vi "Does the Text Fit.vi"(0 "user-specified font":T1, 5 "token string":string, 7 "Capitalize Text":bool) -> (4 "Text Fits":bool)   [LabVIEW 2020, in "Text-Based VI Icon.lvlib"]
uses:
  <vilib>/LabVIEW Icon API/Set Text Icon/Text-Based VI Icon.lvlib
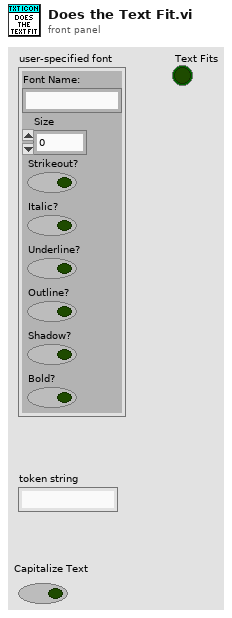
[diagram p1: front panel]
types:
  T1 = cluster{"Font Name:":string, "Size":i16, "Strikeout?":bool, "Italic?":bool, "Underline?":bool, "Outline?":bool, "Shadow?":bool, "Bold?":bool}
  T2 = enum16{"User-specified Font", "Application Font", "System Font", "Dialog Font"}
  T3 = cluster{"left":i16, "top":i16, "right":i16, "bottom":i16}
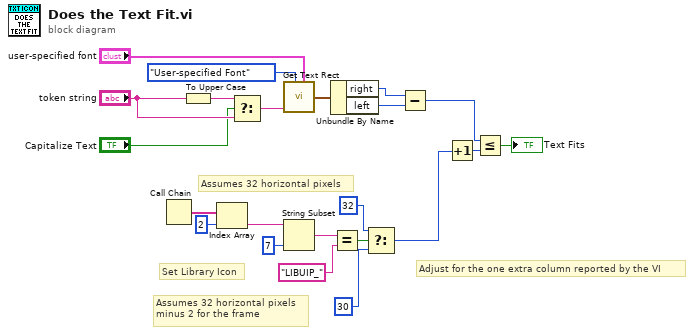
[diagram p0: block diagram]
diagram:
  # "Assumes 32 horizontal pixels\nminus 2 for the frame"
  # "Assumes 32 horizontal pixels"
  # "Set Library Icon"
  # "Adjust for the one extra column reported by the VI"
  n1 = Call Chain() -> (call chain=w10:string[])
  n2 = To Upper Case(1:"token string") -> (0:w14:string)
  n3 = Index Array(array=w10, index=2) -> (element=w8:string)
  n4 = Select(t=w14, s="Capitalize Text", f="token string") -> (s? t:f=w11:string)
  n5 = call <vilib>:"Get Text Rect.vi"("desired font(Application)"=T2."User-specified Font", "text"=w11, "[user-specified font]"="user-specified font") -> ("rect"=w18:T3)  [unwired: 6 in]
  n6 = String Subset(string=w8, length (rest)=7 ("length (rest)")) -> (substring=w6:string)  [unwired: 1 in]
  n7 = Unbundle By Name(w18) -> ("right"=w20:i16, "left"=w21:i16)
  n8 = Equal?(x=w6, y="LIBUIP_") -> (x = y?=w4:bool)
  n9 = Select(t=i16 32, s=w4, f=i16 30) -> (s? t:f=w2:i16)
  n10 = Subtract(x=w20, y=w21) -> (x-y=w22:i16)
  n11 = Increment(x=w2) -> (x+1=w15:i16)
  n12 = Less Or Equal?(x=w22, y=w15) -> (x <= y?=→"Text Fits":bool)
